vi "flattenToString.vi"(8 "error in (no error)":errorcluster, 10 "Record":refnum<class "Record.lvclass">, 11 "Serializer.XML in":refnum<class "Serializer.XML.lvclass">) -> (0 "error out":errorcluster, 2 "Flattened String":string, 3 "Serializer.XML out":refnum<class "Serializer.XML.lvclass">)   [LabVIEW 2017, in "Serializer.Plug-in.lvlib" / "Serializer.XML.lvclass"]
uses:
  Serializer.XML.lvclass
  Record/Record.lvclass
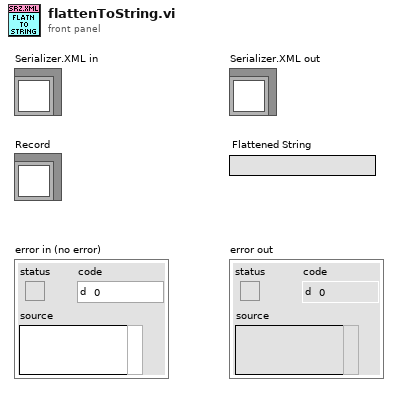
[diagram p1: front panel]
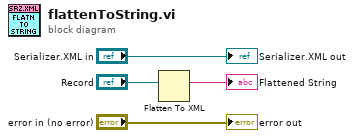
[diagram p0: block diagram]
diagram:
  n1 = Flatten To XML(anything="Record") -> (xml string=→"Flattened String":string)
  "error out" <- "error in (no error)"
  "Serializer.XML out" <- "Serializer.XML in"
